vi "getIntrinsicZk.vi"(8 "error in (no error)":errorcluster, 9 "Field Idx":i32[](array[numeric]), 10 "Filter Type":T1, 11 "OptStateEsti in":refnum<class "OptStateEsti.lvclass">) -> (0 "error out":errorcluster, 2 "Intrinsic Zk":dbl[][](array[numeric]), 3 "OptStateEsti out":refnum<class "OptStateEsti.lvclass">)   [LabVIEW 2016, in "OfcFunc.lvlib" / "OptStateEsti.lvclass"]
doc: "Get the intrinsic zk of specific filter based on the array of field index. The output array shape is nx1."
uses:
  OptStateEsti.lvclass
  StrictDef/FilterType.ctl
  OptStateEsti.lvclass/OptStateEsti.ctl
  MatOper/MatOper.lvclass
  OfcFunc.lvlib
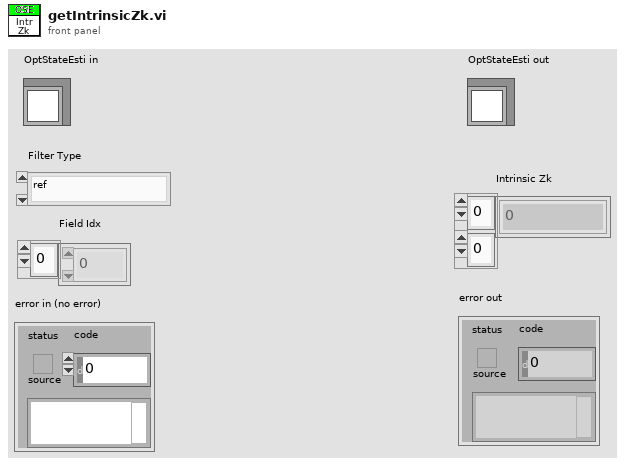
[diagram p1: front panel]
types:
  T1 = typedef "OfcFunc.lvlib/FilterType.ctl" = enum16{"ref", "u", "g", "r", "i", "z", "y"}
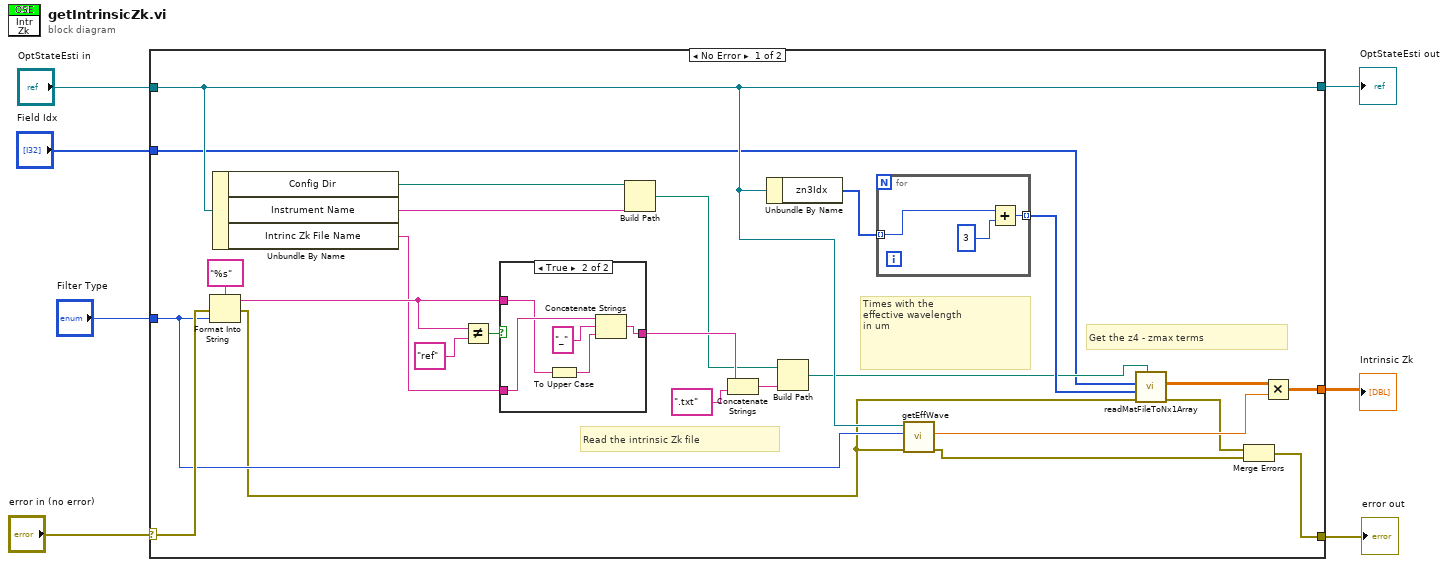
[diagram p0: block diagram]
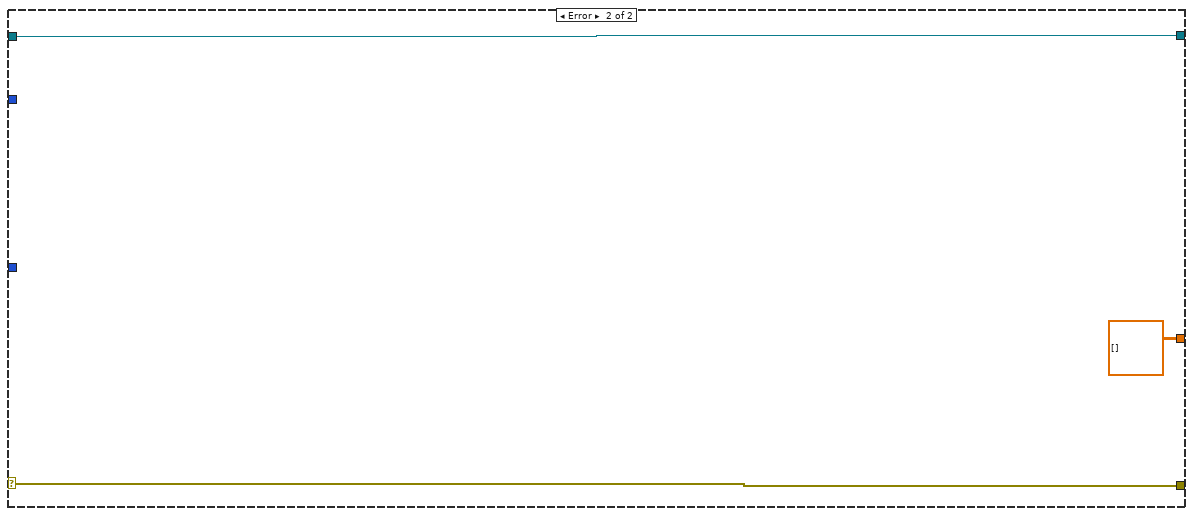
[diagram p3: hidden frame]
diagram:
  n1 = case shown="No Error" "error in (no error)" {
    selector: "error in (no error)" -> [w20 w44]
    tunnel: [w13 w44] -> w6
    tunnel: [w16 w43] -> w5
    tunnel: "OptStateEsti in" -> [w16 w43]
    tunnel: [w25 dbl[][] []] -> w4
    tunnel: "Filter Type" -> [w15 _]
    tunnel: "Field Idx" -> [w8 _]
    frame No Error {
      # "Times with the \neffective wavelength\nin um"
      # "Get the z4 - zmax terms"
      # "Read the intrinsic Zk file"
      n2 = Format Into String(format string="%s", error in=w20, w15) -> (resulting string=w19:string, error out=w14:errorcluster)  [unwired: 1 in]
      n3 = Unbundle By Name(w16) -> ("Config Dir"=w22:path, "Instrument Name"=w28:string, "Intrinc Zk File Name"=w18:string)
      n4 = Not Equal?(x=w19, y="ref") -> (x != y?=w32:bool)
      n5 = case shown="True" w32 {
        tunnel: w18 -> [w36 w41]
        tunnel: [w36 w37] -> w30
        tunnel: w19 -> [_ w39]
        frame False {
        }
        frame True {
          n6 = To Upper Case(1:w39) -> (0:w38:string)
          n7 = Concatenate Strings(w41, "_" ("string"), w38) -> (w37:string)
        }
      }
      n8 = Build Path(base path=w22, name or relative path=w28) -> (appended path=w27:path)
      n9 = Concatenate Strings(w30, ".txt" ("string")) -> (w9:string)
      n10 = Unbundle By Name(w16) -> ("zn3Idx"=w23:i32[])
      n11 = Build Path(base path=w27, name or relative path=w9) -> (appended path=w10:path)
      n12 = for {
        tunnel: w23 -> [w35] mode=indexing
        tunnel: [w34] -> w24 mode=indexing
        n13 = Add(x=w35, y=3) -> (x+y=w34:i32)
      }
      n14 = call "getEffWave.vi"("error in (no error)"=w14, "Filter Type"=w15, "OptStateEsti in"=w16) -> ("error out"=w11:errorcluster, "Effective Wavelength  (um)"=w17:dbl)  [unwired: 6 in, 1 out]
      n15 = call "readMatFileToNx1Array.vi"("Path"=w10, "error in (no error)"=w14, "Index of Column"=w24, "Index of Row"=w8) -> ("error out"=w12:errorcluster, "nx1 Array"=w26:dbl[][])  [unwired: 5 in, 1 out]
      n16 = Merge Errors(w12, w11) -> (w13:errorcluster)
      n17 = Multiply(x=w26, y=w17) -> (x*y=w25:dbl[][])
    }
    frame Error {
    }
  }
  "error out" <- w6
  "OptStateEsti out" <- w5
  "Intrinsic Zk" <- w4
